vi "sub vi - get calibration values v1.vi"() -> (3 "TEMP REF CAL":dbl, 4 "LAB01 (CAL)":T1 {"2 (TN) cal" min=0.0 step=0.01 format="%.2f"; "2 (TL) cal" min=0.0 step=0.01 format="%.2f"; "2 (PF) cal" min=0.0 step=0.01 format="%.2f"; "2 (V) cal" min=0.0 step=0.01 format="%.2f"; "2 (A) cal" min=0.0 step=0.01 format="%.2f"; "1 (TN) cal" min=0.0 step=0.01 format="%.2f"; "1 (TL) cal" min=0.0 step=0.01 format="%.2f"; "1 (PF) cal" min=0.0 step=0.01 format="%.2f"; "1 (V) cal" min=0.0 step=0.01 format="%.2f"; "1  (A) cal" min=0.0 step=0.01 format="%.2f"}, 6 "LAB02 (CAL)":T2 {"2 (TN) cal" min=0.0 step=0.01 format="%.2f"; "2 (TL) cal" min=0.0 step=0.01 format="%.2f"; "2 (PF) cal" min=0.0 step=0.01 format="%.2f"; "2 (V) cal" min=0.0 step=0.01 format="%.2f"; "2 (A) cal" min=0.0 step=0.01 format="%.2f"; "1 (TN) cal" min=0.0 step=0.01 format="%.2f"; "1 (TL) cal" min=0.0 step=0.01 format="%.2f"; "1 (PF) cal" min=0.0 step=0.01 format="%.2f"; "1 (V) cal" min=0.0 step=0.01 format="%.2f"; "1 (A) cal" min=0.0 step=0.01 format="%.2f"}, 8 "LAB03 (CAL)":T1 {"2 (TN) cal" min=0.0 step=0.01 format="%.2f"; "2 (TL) cal" min=0.0 step=0.01 format="%.2f"; "2 (PF) cal" min=0.0 step=0.01 format="%.2f"; "2 (V) cal" min=0.0 step=0.01 format="%.2f"; "2 (A) cal" min=0.0 step=0.01 format="%.2f"; "1 (TN) cal" min=0.0 step=0.01 format="%.2f"; "1 (TL) cal" min=0.0 step=0.01 format="%.2f"; "1 (PF) cal" min=0.0 step=0.01 format="%.2f"; "1 (V) cal" min=0.0 step=0.01 format="%.2f"; "1  (A) cal" min=0.0 step=0.01 format="%.2f"}, 10 "LAB04 (CAL)":T1 {"2 (TN) cal" min=0.0 step=0.01 format="%.2f"; "2 (TL) cal" min=0.0 step=0.01 format="%.2f"; "2 (PF) cal" min=0.0 step=0.01 format="%.2f"; "2 (V) cal" min=0.0 step=0.01 format="%.2f"; "2 (A) cal" min=0.0 step=0.01 format="%.2f"; "1 (TN) cal" min=0.0 step=0.01 format="%.2f"; "1 (TL) cal" min=0.0 step=0.01 format="%.2f"; "1 (PF) cal" min=0.0 step=0.01 format="%.2f"; "1 (V) cal" min=0.0 step=0.01 format="%.2f"; "1  (A) cal" min=0.0 step=0.01 format="%.2f"}, 14 "calibration file error out":errorcluster, 15 "LAB05 (CAL)":T1 {"2 (TN) cal" min=0.0 step=0.01 format="%.2f"; "2 (TL) cal" min=0.0 step=0.01 format="%.2f"; "2 (PF) cal" min=0.0 step=0.01 format="%.2f"; "2 (V) cal" min=0.0 step=0.01 format="%.2f"; "2 (A) cal" min=0.0 step=0.01 format="%.2f"; "1 (TN) cal" min=0.0 step=0.01 format="%.2f"; "1 (TL) cal" min=0.0 step=0.01 format="%.2f"; "1 (PF) cal" min=0.0 step=0.01 format="%.2f"; "1 (V) cal" min=0.0 step=0.01 format="%.2f"; "1  (A) cal" min=0.0 step=0.01 format="%.2f"})   [LabVIEW 2013]
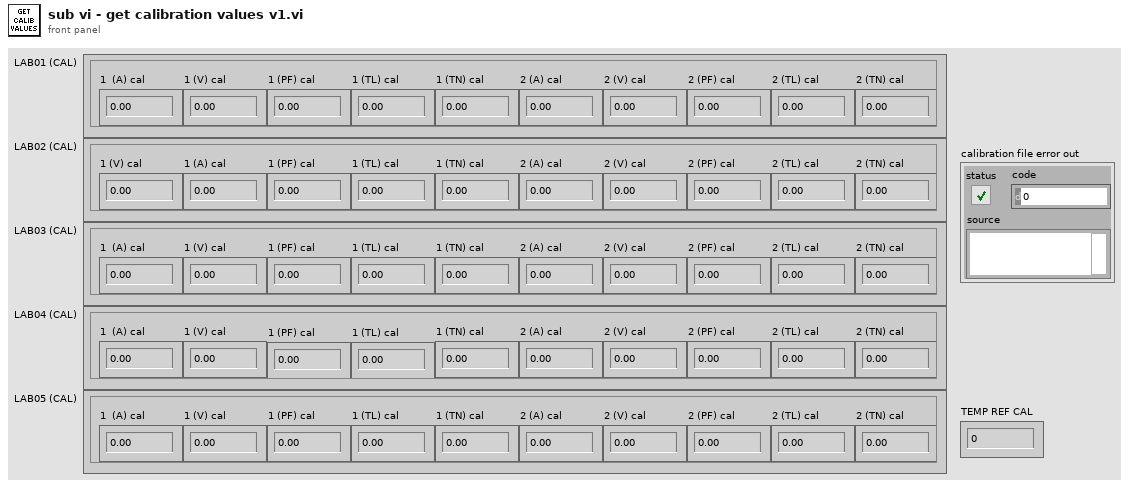
[diagram p1: front panel]
types:
  T1 = cluster{"1  (A) cal":dbl, "1 (V) cal":dbl, "1 (PF) cal":dbl, "1 (TL) cal":dbl, "1 (TN) cal":dbl, "2 (A) cal":dbl, "2 (V) cal":dbl, "2 (PF) cal":dbl, "2 (TL) cal":dbl, "2 (TN) cal":dbl}
  T2 = cluster{"1 (A) cal":dbl, "1 (V) cal":dbl, "1 (PF) cal":dbl, "1 (TL) cal":dbl, "1 (TN) cal":dbl, "2 (A) cal":dbl, "2 (V) cal":dbl, "2 (PF) cal":dbl, "2 (TL) cal":dbl, "2 (TN) cal":dbl}
  T3 = enum16{"open", "replace", "create", "open or create", "replace or create", "replace or create with confirmation"}
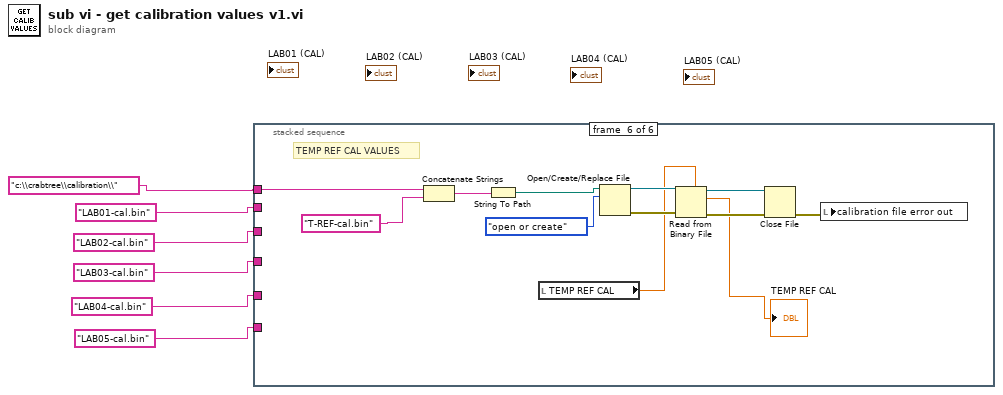
[diagram p0: block diagram]
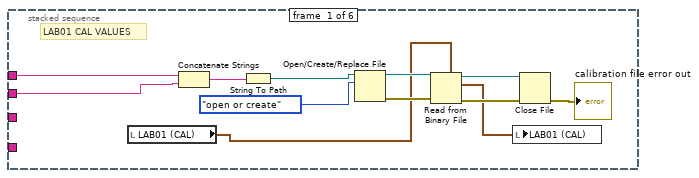
[diagram p2: hidden frame]
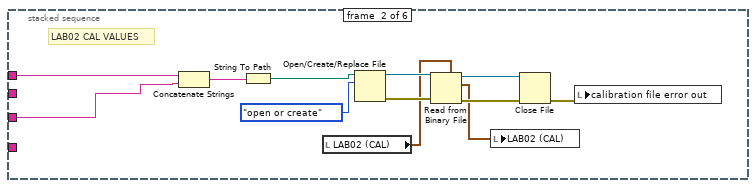
[diagram p3: hidden frame]
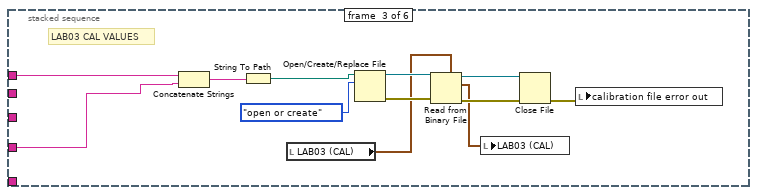
[diagram p4: hidden frame]
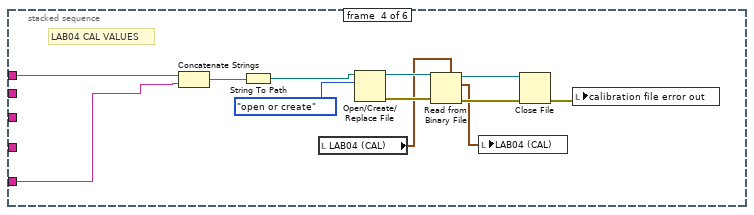
[diagram p5: hidden frame]
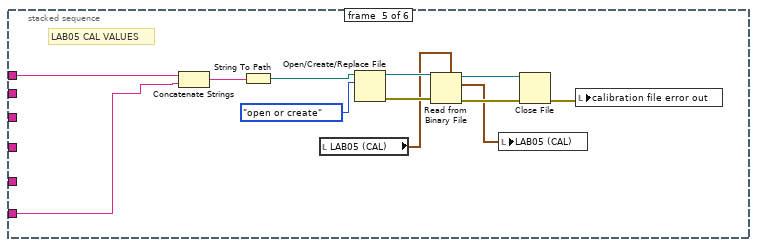
[diagram p6: hidden frame]
diagram:
  n1 = stacked-sequence {
    tunnel: "c:\\crabtree\\calibration\\" -> [w18 w30 w42 w54 w66 w78]
    tunnel: "LAB01-cal.bin" -> [w9 _ _ _ _ _]
    tunnel: "LAB02-cal.bin" -> [_ w21 _ _ _ _]
    tunnel: "LAB03-cal.bin" -> [_ _ w33 _ _ _]
    tunnel: "LAB04-cal.bin" -> [_ _ _ w46 _ _]
    tunnel: "LAB05-cal.bin" -> [_ _ _ _ w57 _]
    frame #0 {
      # "LAB01 CAL VALUES"
      n2 = local read "LAB01 (CAL)"() -> (w8:T1)
      n3 = Concatenate Strings(w18, w9) -> (w17:string)
      n4 = String To Path(string=w17) -> (path=w16:path)
      n5 = Open/Create/Replace File(file path (use dialog)=w16, operation (0:open)=T3."open or create") -> (refnum out=w15:refnum<file>, error out=w14:errorcluster)  [unwired: 4 in, 1 out]
      n6 = Read from Binary File(5:w8, 8:w14, 11:w15) -> (0:w12:errorcluster, 2:w7:T1, 3:w13:refnum<file>)  [unwired: 3 in, 1 out]
      n7 = local write "LAB01 (CAL)"(w7) -> ()
      n8 = Close File(refnum=w13, error in=w12) -> (error out=→"calibration file error out":errorcluster)  [unwired: 1 out]
    }
    frame #1 {
      # "LAB02 CAL VALUES"
      n9 = Concatenate Strings(w30, w21) -> (w29:string)
      n10 = String To Path(string=w29) -> (path=w28:path)
      n11 = local read "LAB02 (CAL)"() -> (w20:T2)
      n12 = Open/Create/Replace File(file path (use dialog)=w28, operation (0:open)=T3."open or create") -> (refnum out=w27:refnum<file>, error out=w26:errorcluster)  [unwired: 4 in, 1 out]
      n13 = Read from Binary File(5:w20, 8:w26, 11:w27) -> (0:w24:errorcluster, 2:w19:T2, 3:w25:refnum<file>)  [unwired: 3 in, 1 out]
      n14 = local write "LAB02 (CAL)"(w19) -> ()
      n15 = Close File(refnum=w25, error in=w24) -> (error out=w22:errorcluster)  [unwired: 1 out]
      n16 = local write "calibration file error out"(w22) -> ()
    }
    frame #2 {
      # "LAB03 CAL VALUES"
      n17 = Concatenate Strings(w42, w33) -> (w41:string)
      n18 = String To Path(string=w41) -> (path=w40:path)
      n19 = local read "LAB03 (CAL)"() -> (w32:T1)
      n20 = Open/Create/Replace File(file path (use dialog)=w40, operation (0:open)=T3."open or create") -> (refnum out=w39:refnum<file>, error out=w38:errorcluster)  [unwired: 4 in, 1 out]
      n21 = Read from Binary File(5:w32, 8:w38, 11:w39) -> (0:w36:errorcluster, 2:w31:T1, 3:w37:refnum<file>)  [unwired: 3 in, 1 out]
      n22 = local write "LAB03 (CAL)"(w31) -> ()
      n23 = Close File(refnum=w37, error in=w36) -> (error out=w34:errorcluster)  [unwired: 1 out]
      n24 = local write "calibration file error out"(w34) -> ()
    }
    frame #3 {
      # "LAB04 CAL VALUES"
      n25 = Concatenate Strings(w54, w46) -> (w53:string)
      n26 = String To Path(string=w53) -> (path=w52:path)
      n27 = local read "LAB04 (CAL)"() -> (w44:T1)
      n28 = Open/Create/Replace File(file path (use dialog)=w52, operation (0:open)=T3."open or create") -> (refnum out=w51:refnum<file>, error out=w50:errorcluster)  [unwired: 4 in, 1 out]
      n29 = Read from Binary File(5:w44, 8:w50, 11:w51) -> (0:w48:errorcluster, 2:w43:T1, 3:w49:refnum<file>)  [unwired: 3 in, 1 out]
      n30 = local write "LAB04 (CAL)"(w43) -> ()
      n31 = Close File(refnum=w49, error in=w48) -> (error out=w47:errorcluster)  [unwired: 1 out]
      n32 = local write "calibration file error out"(w47) -> ()
    }
    frame #4 {
      # "LAB05 CAL VALUES"
      n33 = Concatenate Strings(w66, w57) -> (w65:string)
      n34 = String To Path(string=w65) -> (path=w64:path)
      n35 = local read "LAB05 (CAL)"() -> (w56:T1)
      n36 = Open/Create/Replace File(file path (use dialog)=w64, operation (0:open)=T3."open or create") -> (refnum out=w63:refnum<file>, error out=w62:errorcluster)  [unwired: 4 in, 1 out]
      n37 = Read from Binary File(5:w56, 8:w62, 11:w63) -> (0:w60:errorcluster, 2:w55:T1, 3:w61:refnum<file>)  [unwired: 3 in, 1 out]
      n38 = local write "LAB05 (CAL)"(w55) -> ()
      n39 = Close File(refnum=w61, error in=w60) -> (error out=w58:errorcluster)  [unwired: 1 out]
      n40 = local write "calibration file error out"(w58) -> ()
    }
    frame #5 {
      # "TEMP REF CAL VALUES"
      n41 = Concatenate Strings(w78, "T-REF-cal.bin") -> (w77:string)
      n42 = String To Path(string=w77) -> (path=w76:path)
      n43 = local read "TEMP REF CAL"() -> (w68:dbl)
      n44 = Open/Create/Replace File(file path (use dialog)=w76, operation (0:open)=T3."open or create") -> (refnum out=w75:refnum<file>, error out=w74:errorcluster)  [unwired: 4 in, 1 out]
      n45 = Read from Binary File(5:w68, 8:w74, 11:w75) -> (0:w72:errorcluster, 2:→"TEMP REF CAL":dbl, 3:w73:refnum<file>)  [unwired: 3 in, 1 out]
      n46 = Close File(refnum=w73, error in=w72) -> (error out=w70:errorcluster)  [unwired: 1 out]
      n47 = local write "calibration file error out"(w70) -> ()
    }
  }
